vi "Default Configuration.vi"() -> (3 "Default Configuration":T1={"Common"={"Period (s)"=0.001, "T0 (ns)"=0, "ClockID"=0, "Priority"=100, "Processor"=-2}, "Quotient"=100} {"Common"."Period (s)" format="%#_13g"})   [LabVIEW 2021, in "CIFTemplatePlugin.lvclass"]
uses:
  CIFTemplatePlugin.lvclass
  Shared/Typedef/Configuration.ctl
  CIFCore/CIFCoreCommon/Typedef/Common Plugin Configuration.ctl
  CIFCore/CIFCoreCommon/CIFCoreCommon.lvlib
  Shared/CIFTemplatePluginShared.lvlib
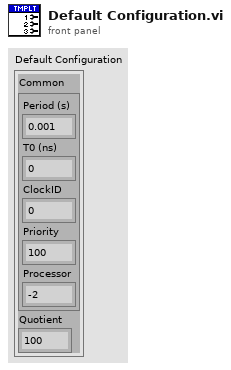
[diagram p1: front panel]
types:
  T1 = typedef "CIFTemplatePluginShared.lvlib/Configuration.ctl" = cluster{"Common":T2, "Quotient":u32}
  T2 = typedef "CIFCoreCommon.lvlib/Common Plugin Configuration.ctl" = cluster{"Period (s)":dbl, "T0 (ns)":u64, "ClockID":u8, "Priority":i32, "Processor":i32}
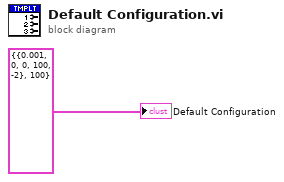
[diagram p0: block diagram]
diagram:
  "Default Configuration" <- T1 {"Common"={"Period (s)"=0.001, "T0 (ns)"=0, "ClockID"=0, "Priority"=100, "Processor"=-2}, "Quotient"=100} ("Template Configuration")
